vi "Launch Wrapper.vi"(0 "Controller in":refnum<class "Controller.lvclass">) -> (14 "Controller out":refnum<class "Controller.lvclass">, 19 "error out":errorcluster)   [LabVIEW 2014, in "Controller.lvlib" / "Controller.lvclass"]
uses:
  Controller.lvclass
  <vilib>/ActorFramework/Actor/Actor.lvclass
  Controls/Notifier Enum.ctl
  <vilib>/Utility/config.llb/NI_LVConfig.lvlib
  <vilib>/Utility/config.llb/Read Key (Boolean).vi
  <vilib>/Utility/config.llb/Read Key (I32).vi
  reusable/Switch/Switch.lvclass
  <vilib>/NI_Real-Time Target Support.lvlib
  Messages/Update Filter State Params/Update Filter Cycle Params MSG.lvclass
  Messages/Change Filter State/Change Filter State.lvclass
  <vilib>/ActorFramework/Message Enqueuer/Message Enqueuer.lvclass
  xGlobal Data.vi
  reusable/Session APIs/Session Log/System Log.lvclass
  <userlib>/_Session Fwk/Session - Root.lvclass
  Messages/Change Inlet MSG/Change Inlet MSG.lvclass
  <vilib>/Utility/config.llb/Read Key (String).vi
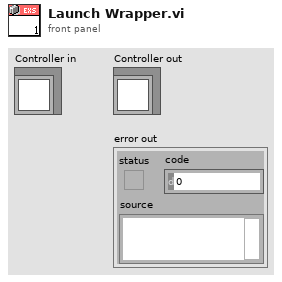
[diagram p1: front panel]
types:
  T1 = typedef "Notifier Enum.ctl" = enum16{"Initialize", "Get", "Set", "Close"}
  T2 = typedef "NI_LVConfig.lvlib/Config Data RefNum.ctl" = refnum<k1>
  T3 = typedef "Session - Root.lvclass/Session Handle.ctl" = refnum<data-value>
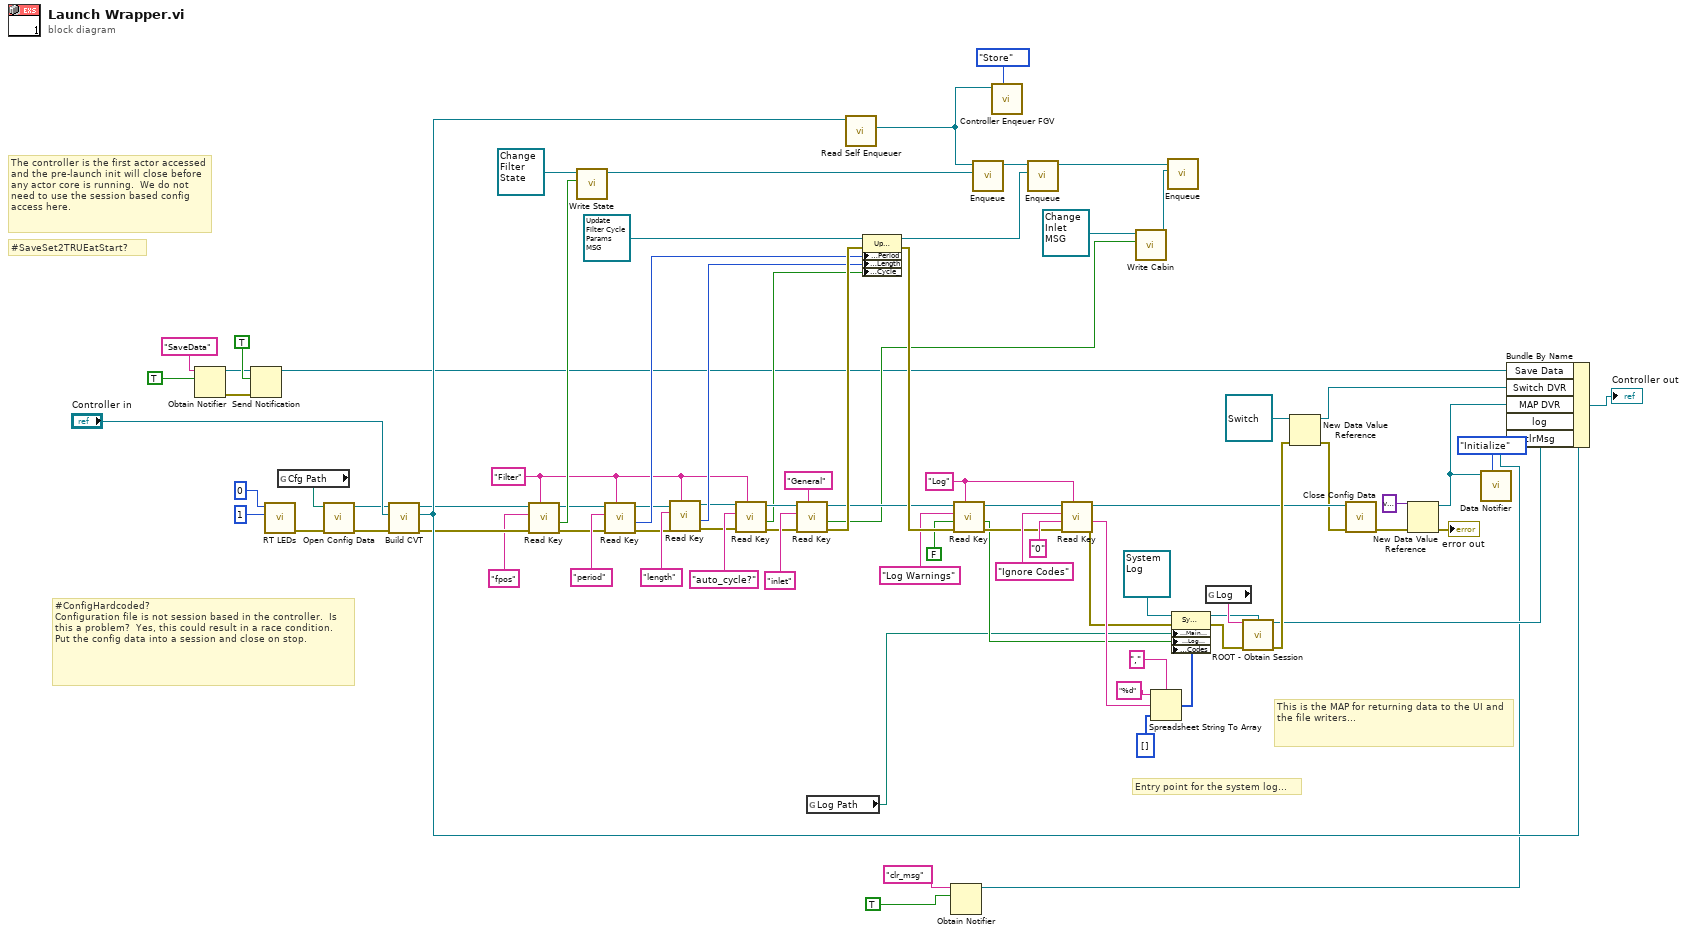
[diagram p0: block diagram]
diagram:
  w71 = "Log" ("section")
  w26 = "Filter" ("section")
  # "Entry point for the system log..."
  # "This is the MAP for returning data to the UI and the file writers..."
  # "#ConfigHardcoded?\nConfiguration file is not session based in the controller.  Is this a problem?  Yes, this could result in a race condition.  Put the config data into a session and close on stop."
  # "#SaveSet2TRUEatStart?"
  # "The controller is the first actor accessed and the pre-launch init will close before any actor core is running.  We do not need to use the session based config access here."
  n1 = Obtain Notifier(name (unnamed)="SaveData", notification data type=TRUE) -> (notifier out=w7:refnum<notifier>, error out=w8:errorcluster)  [unwired: 2 in, 1 out]
  n2 = Send Notification(notification=TRUE, notifier=w7, error in (no error)=w8) -> (notifier out=w10:refnum<notifier>)  [unwired: 1 out]
  n3 = call <vilib>:"RT LEDs.vi"("State"=1, "LED Num"=0) -> ("error out"=w21:errorcluster)  [unwired: 4 in, 1 out]
  n4 = global read "xGlobal Data.vi" "Cfg Path"() -> (w36:path)
  n5 = call <vilib>:"Open Config Data.vi"("error in (no error)"=w21, "configuration file path"=w36) -> ("error out"=w52:errorcluster, "refnum"=w51:T2)  [unwired: 7 in, 1 out]
  n6 = call "Build CVT.vi"("Error In"=w52, "Controller in"="Controller in", "CfgRef"=w51) -> ("Error Out"=w54:errorcluster, "Controller out"=w64:refnum<class "Controller.lvclass">, "refnum out"=w53:T2)  [unwired: 6 in]
  n7 = call-poly <vilib>:"Read Key.vi"("section"=w26, "error in (no error)"=w54, "key"="fpos", "refnum"=w53) -> ("error out"=w14:errorcluster, "value"=w37:bool, "refnum out"=w13:T2)  [unwired: 4 in, 1 out]
  n8 = call "Write State.vi"("State"=w37, "Change Filter State in"=refnum<class "Change Filter State.lvclass"> refnum ("Controller.lvlib:Change Filter State MSG")) -> ("Change Filter State out"=w32:refnum<class "Change Filter State.lvclass">)  [unwired: 8 in, 1 out]
  n9 = call-poly <vilib>:"Read Key.vi"("section"=w26, "error in (no error)"=w14, "key"="period", "refnum"=w13) -> ("error out"=w17:errorcluster, "value"=w48:i32, "refnum out"=w16:T2)  [unwired: 4 in, 1 out]
  n10 = call-poly <vilib>:"Read Key.vi"("section"=w26, "error in (no error)"=w17, "key"="length", "refnum"=w16) -> ("error out"=w25:errorcluster, "value"=w49:i32, "refnum out"=w24:T2)  [unwired: 4 in, 1 out]
  n11 = call-poly <vilib>:"Read Key.vi"("section"=w26, "error in (no error)"=w25, "key"="auto_cycle?", "refnum"=w24) -> ("error out"=w56:errorcluster, "value"=w50:bool, "refnum out"=w55:T2)  [unwired: 4 in, 1 out]
  n12 = call-poly <vilib>:"Read Key.vi"("section"="General", "error in (no error)"=w56, "key"="inlet", "refnum"=w55) -> ("error out"=w81:errorcluster, "value"=w61:bool, "refnum out"=w65:T2)  [unwired: 4 in, 1 out]
  n13 = global read "xGlobal Data.vi" "Log Path"() -> (w46:path)
  n14 = call <vilib>:"Read Self Enqueuer.vi"("Actor"=w64) -> ("Self Enqueuer"=w31:refnum<class "Message Enqueuer.lvclass">)  [unwired: 10 in]
  n15 = property class="Update Filter Cycle Params"(reference=refnum<class "Update Filter Cycle Params MSG.lvclass"> refnum ("Controller.lvlib:Update Filter Cycle Params"), error in=w81, "Accessors:Period"=w48, "Accessors:Length"=w49, "Accessors:Cycle_"=w50) -> (reference out=w34:refnum<class "Update Filter Cycle Params MSG.lvclass">, error out=w82:errorcluster)
  n16 = Obtain Notifier(name (unnamed)="clr_msg", notification data type=TRUE) -> (notifier out=w1:refnum<notifier>)  [unwired: 2 in, 2 out]
  n17 = call-poly <vilib>:"Read Key.vi"("section"=w71, "error in (no error)"=w82, "default value"=FALSE, "key"="Log Warnings", "refnum"=w65) -> ("error out"=w70:errorcluster, "value"=w68:bool, "refnum out"=w69:T2)  [unwired: 3 in, 1 out]
  n18 = call <vilib>:"Enqueue.vi"("Message"=w32, "Message Enqueuer in"=w31) -> ("Message Enqueuer out"=w33:refnum<class "Message Enqueuer.lvclass">)  [unwired: 8 in, 1 out]
  n19 = call "Controller Enqeuer FGV.vi"("State"=enum16{"Store", "Send MSG"}."Store", "Enqueuer"=w31) -> ()  [unwired: 9 in, 1 out]
  n20 = call <vilib>:"Enqueue.vi"("Message"=w34, "Message Enqueuer in"=w33) -> ("Message Enqueuer out"=w59:refnum<class "Message Enqueuer.lvclass">)  [unwired: 8 in, 1 out]
  n21 = call-poly <vilib>:"Read Key.vi"("section"=w71, "error in (no error)"=w70, "default value"="0", "key"="Ignore Codes", "refnum"=w69) -> ("error out"=w74:errorcluster, "value"=w76:string, "refnum out"=w73:T2)  [unwired: 3 in, 1 out]
  n22 = call "Write Cabin.vi"("Cabin"=w61, "Change Inlet MSG in"=refnum<class "Change Inlet MSG.lvclass"> refnum ("Controller.lvlib:Change Inlet MSG.lvclass")) -> ("Change Inlet MSG out"=w62:refnum<class "Change Inlet MSG.lvclass">)  [unwired: 8 in, 1 out]
  n23 = Spreadsheet String To Array(delimiter (Tab)=",", format string="%d", spreadsheet string=w76, array type (2D Dbl)=i32[] []) -> (array=w80:i32[])
  n24 = call <vilib>:"Enqueue.vi"("Message"=w62, "Message Enqueuer in"=w59) -> ()  [unwired: 8 in, 2 out]
  n25 = property class="Sys Log"(reference=refnum<class "System Log.lvclass"> refnum ("Sys Log"), error in=w74, "Accessors:Main Path"=w46, "Accessors:Log Warnings_"=w68, "Accessors:Codes"=w80) -> (reference out=w44:refnum<class "System Log.lvclass">, error out=w42:errorcluster)
  n26 = global read "xGlobal Data.vi" "Log"() -> (w45:string)
  n27 = call <userlib>:"ROOT - Obtain Session.vi"("Session Name ()"=w45, "OBJ - Session"=w44, "error in (no error)"=w42) -> ("Session Handle"=w47:T3, "error out"=w83:errorcluster)  [unwired: 10 in, 1 out]
  n28 = New Data Value Reference(data value=refnum<class "Switch.lvclass"> refnum ("Switch"), error in=w83) -> (data value reference=w35:refnum<data-value>, error out=w22:errorcluster)
  n29 = call <vilib>:"Close Config Data.vi"("error in (no error)"=w22, "refnum"=w73) -> ("error out"=w40:errorcluster)  [unwired: 8 in, 1 out]
  n30 = New Data Value Reference(data value=variant, error in=w40) -> (data value reference=w38:refnum<data-value>, error out=→"error out":errorcluster)
  n31 = call "Data Notifier.vi"("State"=Notifier_Enum."Initialize", "MAP DVR"=w38) -> ()  [unwired: 8 in, 2 out]
  n32 = Bundle By Name(cluster=w64, "Save Data"=w10, "Switch DVR"=w35, "MAP DVR"=w38, "log"=w47, "clrMsg"=w1) -> (→"Controller out":refnum<class "Controller.lvclass">)
